vi "Boolean Logic.vi"() -> ()   [LabVIEW 2019]
panel:
  out "C":bool
  in  "B":bool
  in  "A":bool
  in  "Choice":bool
  out "s? t:f":dbl
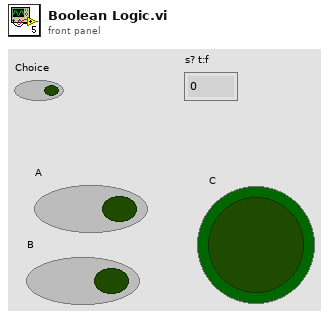
[diagram p1: front panel]
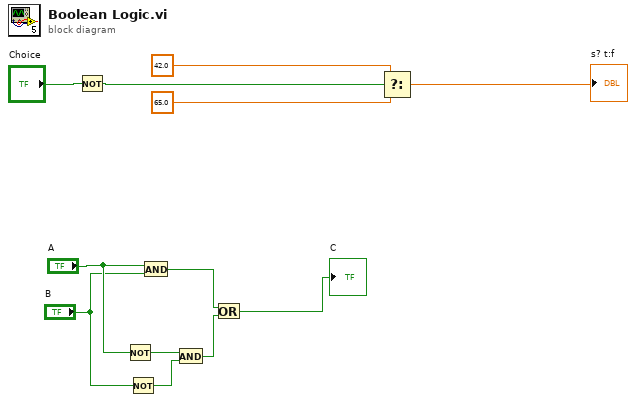
[diagram p0: block diagram]
diagram:
  n1 = Not(x="Choice") -> (.not. x?=w8:bool)
  n2 = Not(x="A") -> (.not. x?=w2:bool)
  n3 = Not(x="B") -> (.not. x?=w1:bool)
  n4 = And(x="A", y="B") -> (x .and. y?=w4:bool)
  n5 = And(x=w2, y=w1) -> (x .and. y?=w5:bool)
  n6 = Or(x=w4, y=w5) -> (x .or. y?=→"C":bool)
  n7 = Select(t=42.0, s=w8, f=65.0) -> (s? t:f=→"s? t:f":dbl)
